vi "SP Initialize Display.vi"(8 "error in (no error)":errorcluster, 10 "Visible? (F)":bool, 11 "Plot References":refnum<vi>[](array[refnum])) -> (0 "error out":errorcluster)   [LabVIEW 2011]
uses:
  TypeDefs/SP Plot Cluster Object.ctl
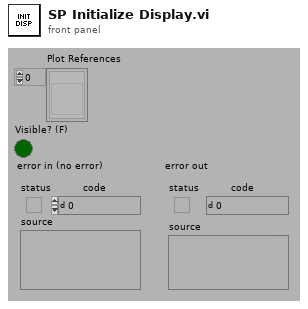
[diagram p1: front panel]
types:
  T1 = typedef "SP Plot Cluster Object.ctl" = enum16{"Plot", "CH Reference", "CH Label", "Start Label", "Stop Label", "Units Label", "Selected?", "CH Markers"}
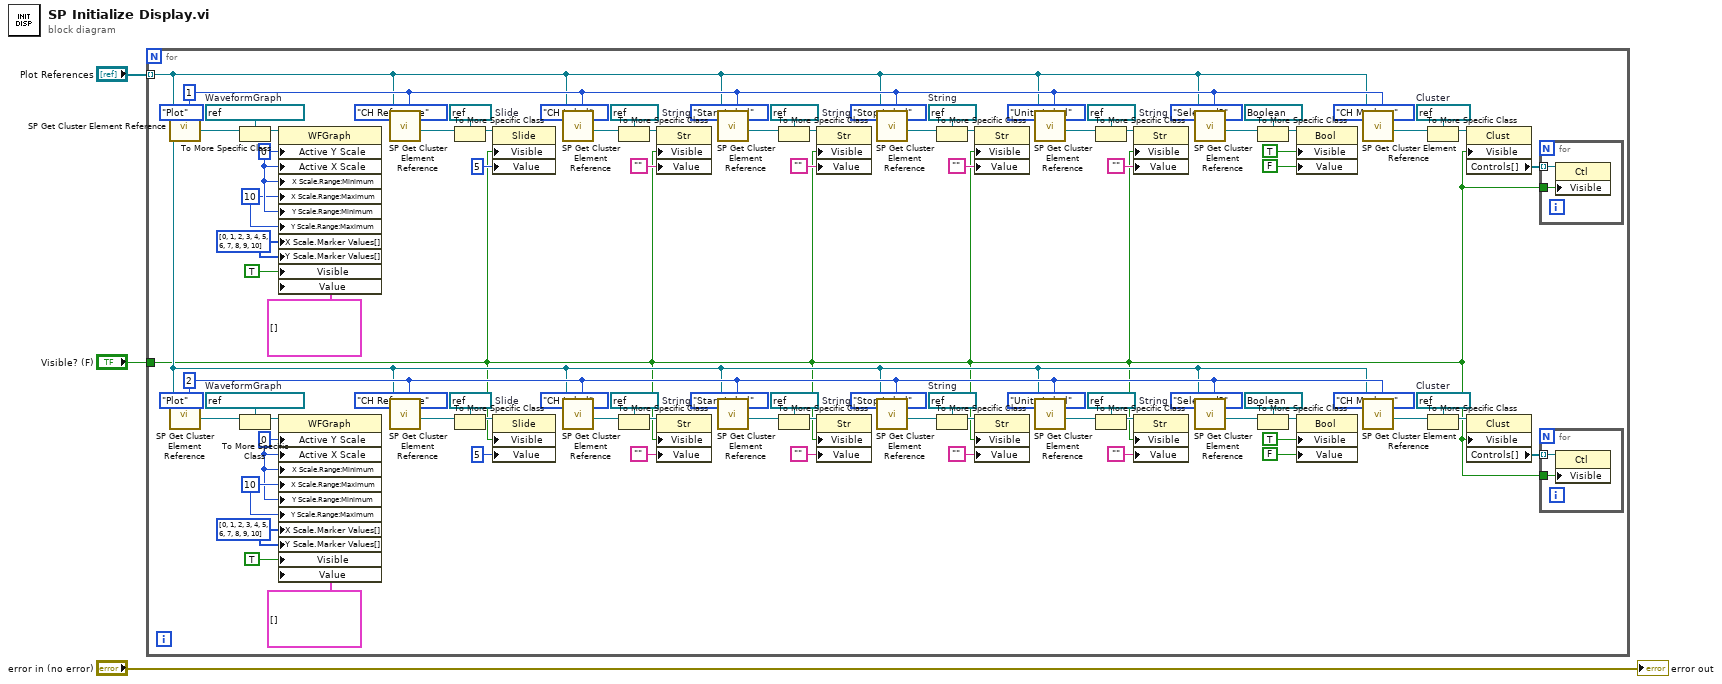
[diagram p0: block diagram]
diagram:
  n1 = for {
    tunnel: "Plot References" -> [w21] mode=indexing
    tunnel: "Visible? (F)" -> [w4]
    w12 = i8[] [0, 1, 2, 3, 4, 5, 6, 7, 8, 9, 10] ("X Scale.Marker Values[]")
    w11 = i8 10 ("X Scale.Range:Maximum")
    w10 = i8 0 ("Active Y Scale")
    w15 = i8[] [0, 1, 2, 3, 4, 5, 6, 7, 8, 9, 10] ("X Scale.Marker Values[]")
    w16 = i8 10 ("X Scale.Range:Maximum")
    w17 = i8 0 ("Active Y Scale")
    w59 = refnum<vi> refnum  # Cluster
    w46 = refnum<vi> refnum  # String
    w43 = refnum<vi> refnum  # String
    w36 = refnum<vi> refnum  # String
    w33 = refnum<vi> refnum  # String
    w26 = refnum<vi> refnum  # Slide
    w23 = refnum<vi> refnum  # WaveformGraph
    w58 = 2 ("Channel")
    w60 = refnum<vi> refnum  # Cluster
    w73 = refnum<vi> refnum  # String
    w76 = refnum<vi> refnum  # String
    w83 = refnum<vi> refnum  # String
    w86 = refnum<vi> refnum  # String
    w93 = refnum<vi> refnum  # Slide
    w96 = refnum<vi> refnum  # WaveformGraph
    w61 = 1 ("Channel")
    n2 = call "SP Get Cluster Element Reference.vi"("Channel"=w61, "Element"=SP_Plot_Cluster_Object."Plot", "Plot Reference"=w21) -> ("Element Reference"=w95:refnum<vi>)  [unwired: 6 out]
    n3 = call "SP Get Cluster Element Reference.vi"("Channel"=w58, "Element"=SP_Plot_Cluster_Object."Plot", "Plot Reference"=w21) -> ("Element Reference"=w24:refnum<vi>)  [unwired: 6 out]
    n4 = To More Specific Class(target class=w96, reference=w95) -> (specific class reference=w18:refnum<vi>)  [unwired: 1 in, 1 out]
    n5 = To More Specific Class(target class=w23, reference=w24) -> (specific class reference=w9:refnum<vi>)  [unwired: 1 in, 1 out]
    n6 = property class="WFGraph"(reference=w18, "Active Y Scale"=w17, "Active X Scale"=w17, "X Scale.Range:Minimum"=w17, "X Scale.Range:Maximum"=w16, "Y Scale.Range:Minimum"=w17, "Y Scale.Range:Maximum"=w16, "X Scale.Marker Values[]"=w15, "Y Scale.Marker Values[]"=w15, "Visible"=TRUE, "Value"=cluster{"X":dbl[], "Y":dbl[]}[] [] ("appended array")) -> ()  [unwired: 1 in, 2 out]
    n7 = property class="WFGraph"(reference=w9, "Active Y Scale"=w10, "Active X Scale"=w10, "X Scale.Range:Minimum"=w10, "X Scale.Range:Maximum"=w11, "Y Scale.Range:Minimum"=w10, "Y Scale.Range:Maximum"=w11, "X Scale.Marker Values[]"=w12, "Y Scale.Marker Values[]"=w12, "Visible"=TRUE, "Value"=cluster{"X":dbl[], "Y":dbl[]}[] [] ("appended array")) -> ()  [unwired: 1 in, 2 out]
    n8 = call "SP Get Cluster Element Reference.vi"("Channel"=w61, "Element"=SP_Plot_Cluster_Object."CH Reference", "Plot Reference"=w21) -> ("Element Reference"=w92:refnum<vi>)  [unwired: 6 out]
    n9 = call "SP Get Cluster Element Reference.vi"("Channel"=w58, "Element"=SP_Plot_Cluster_Object."CH Reference", "Plot Reference"=w21) -> ("Element Reference"=w27:refnum<vi>)  [unwired: 6 out]
    n10 = To More Specific Class(target class=w93, reference=w92) -> (specific class reference=w91:refnum<vi>)  [unwired: 1 in, 1 out]
    n11 = To More Specific Class(target class=w26, reference=w27) -> (specific class reference=w28:refnum<vi>)  [unwired: 1 in, 1 out]
    n12 = property class="Slide"(reference=w91, "Visible"=w4, "Value"=5) -> ()  [unwired: 1 in, 2 out]
    n13 = property class="Slide"(reference=w28, "Visible"=w4, "Value"=5) -> ()  [unwired: 1 in, 2 out]
    n14 = call "SP Get Cluster Element Reference.vi"("Channel"=w61, "Element"=SP_Plot_Cluster_Object."CH Label", "Plot Reference"=w21) -> ("Element Reference"=w88:refnum<vi>)  [unwired: 6 out]
    n15 = call "SP Get Cluster Element Reference.vi"("Channel"=w58, "Element"=SP_Plot_Cluster_Object."CH Label", "Plot Reference"=w21) -> ("Element Reference"=w31:refnum<vi>)  [unwired: 6 out]
    n16 = To More Specific Class(target class=w86, reference=w88) -> (specific class reference=w89:refnum<vi>)  [unwired: 1 in, 1 out]
    n17 = To More Specific Class(target class=w33, reference=w31) -> (specific class reference=w30:refnum<vi>)  [unwired: 1 in, 1 out]
    n18 = property class="Str"(reference=w89, "Visible"=w4, "Value"="") -> ()  [unwired: 1 in, 2 out]
    n19 = property class="Str"(reference=w30, "Visible"=w4, "Value"="") -> ()  [unwired: 1 in, 2 out]
    n20 = call "SP Get Cluster Element Reference.vi"("Channel"=w61, "Element"=SP_Plot_Cluster_Object."Start Label", "Plot Reference"=w21) -> ("Element Reference"=w82:refnum<vi>)  [unwired: 6 out]
    n21 = call "SP Get Cluster Element Reference.vi"("Channel"=w58, "Element"=SP_Plot_Cluster_Object."Start Label", "Plot Reference"=w21) -> ("Element Reference"=w37:refnum<vi>)  [unwired: 6 out]
    n22 = To More Specific Class(target class=w83, reference=w82) -> (specific class reference=w81:refnum<vi>)  [unwired: 1 in, 1 out]
    n23 = To More Specific Class(target class=w36, reference=w37) -> (specific class reference=w38:refnum<vi>)  [unwired: 1 in, 1 out]
    n24 = property class="Str"(reference=w81, "Visible"=w4, "Value"="") -> ()  [unwired: 1 in, 2 out]
    n25 = property class="Str"(reference=w38, "Visible"=w4, "Value"="") -> ()  [unwired: 1 in, 2 out]
    n26 = call "SP Get Cluster Element Reference.vi"("Channel"=w61, "Element"=SP_Plot_Cluster_Object."Stop Label", "Plot Reference"=w21) -> ("Element Reference"=w77:refnum<vi>)  [unwired: 6 out]
    n27 = call "SP Get Cluster Element Reference.vi"("Channel"=w58, "Element"=SP_Plot_Cluster_Object."Stop Label", "Plot Reference"=w21) -> ("Element Reference"=w42:refnum<vi>)  [unwired: 6 out]
    n28 = To More Specific Class(target class=w76, reference=w77) -> (specific class reference=w78:refnum<vi>)  [unwired: 1 in, 1 out]
    n29 = To More Specific Class(target class=w43, reference=w42) -> (specific class reference=w41:refnum<vi>)  [unwired: 1 in, 1 out]
    n30 = property class="Str"(reference=w78, "Visible"=w4, "Value"="") -> ()  [unwired: 1 in, 2 out]
    n31 = property class="Str"(reference=w41, "Visible"=w4, "Value"="") -> ()  [unwired: 1 in, 2 out]
    n32 = call "SP Get Cluster Element Reference.vi"("Channel"=w61, "Element"=SP_Plot_Cluster_Object."Units Label", "Plot Reference"=w21) -> ("Element Reference"=w72:refnum<vi>)  [unwired: 6 out]
    n33 = call "SP Get Cluster Element Reference.vi"("Channel"=w58, "Element"=SP_Plot_Cluster_Object."Units Label", "Plot Reference"=w21) -> ("Element Reference"=w47:refnum<vi>)  [unwired: 6 out]
    n34 = To More Specific Class(target class=w73, reference=w72) -> (specific class reference=w71:refnum<vi>)  [unwired: 1 in, 1 out]
    n35 = To More Specific Class(target class=w46, reference=w47) -> (specific class reference=w48:refnum<vi>)  [unwired: 1 in, 1 out]
    n36 = property class="Str"(reference=w71, "Visible"=w4, "Value"="") -> ()  [unwired: 1 in, 2 out]
    n37 = property class="Str"(reference=w48, "Visible"=w4, "Value"="") -> ()  [unwired: 1 in, 2 out]
    n38 = call "SP Get Cluster Element Reference.vi"("Channel"=w61, "Element"=SP_Plot_Cluster_Object."Selected?", "Plot Reference"=w21) -> ("Element Reference"=w67:refnum<vi>)  [unwired: 6 out]
    n39 = call "SP Get Cluster Element Reference.vi"("Channel"=w58, "Element"=SP_Plot_Cluster_Object."Selected?", "Plot Reference"=w21) -> ("Element Reference"=w52:refnum<vi>)  [unwired: 6 out]
    n40 = To More Specific Class(target class=refnum<vi> refnum ("Selected? Ref"), reference=w67) -> (specific class reference=w68:refnum<vi>)  [unwired: 1 in, 1 out]
    n41 = To More Specific Class(target class=refnum<vi> refnum ("Selected? Ref"), reference=w52) -> (specific class reference=w51:refnum<vi>)  [unwired: 1 in, 1 out]
    n42 = property class="Bool"(reference=w68, "Visible"=TRUE, "Value"=FALSE) -> ()  [unwired: 1 in, 2 out]
    n43 = property class="Bool"(reference=w51, "Visible"=TRUE, "Value"=FALSE) -> ()  [unwired: 1 in, 2 out]
    n44 = call "SP Get Cluster Element Reference.vi"("Channel"=w61, "Element"=SP_Plot_Cluster_Object."CH Markers", "Plot Reference"=w21) -> ("Element Reference"=w64:refnum<vi>)  [unwired: 6 out]
    n45 = call "SP Get Cluster Element Reference.vi"("Channel"=w58, "Element"=SP_Plot_Cluster_Object."CH Markers", "Plot Reference"=w21) -> ("Element Reference"=w55:refnum<vi>)  [unwired: 6 out]
    n46 = To More Specific Class(target class=w60, reference=w64) -> (specific class reference=w63:refnum<vi>)  [unwired: 1 in, 1 out]
    n47 = To More Specific Class(target class=w59, reference=w55) -> (specific class reference=w56:refnum<vi>)  [unwired: 1 in, 1 out]
    n48 = property class="Clust"(reference=w63, "Visible"=w4) -> ("Controls[]"=w6:refnum<vi>[])  [unwired: 1 in, 2 out]
    n49 = property class="Clust"(reference=w56, "Visible"=w4) -> ("Controls[]"=w5:refnum<vi>[])  [unwired: 1 in, 2 out]
    n50 = for {
      tunnel: w6 -> [w101] mode=indexing
      tunnel: w4 -> [w100]
      n51 = property class="Ctl"(reference=w101, "Visible"=w100) -> ()  [unwired: 1 in, 2 out]
    }
    n52 = for {
      tunnel: w5 -> [w99] mode=indexing
      tunnel: w4 -> [w98]
      n53 = property class="Ctl"(reference=w99, "Visible"=w98) -> ()  [unwired: 1 in, 2 out]
    }
  }
  "error out" <- "error in (no error)"
